vi "Write status_state.vi"(8 "error in (no error)":errorcluster, 10 "state":T1=enum."configure", 11 "MB_TCP in":refnum<class "MB_TCP.lvclass">) -> (0 "error out":errorcluster, 3 "MB_TCP out":refnum<class "MB_TCP.lvclass">)   [LabVIEW 2021, in "MB_TCP.lvclass"]
uses:
  MB_TCP.lvclass
  MB_TCP_State.ctl
  MB_TCP.lvclass/MB_TCP.ctl
  Eth Status/Eth Status.lvlib
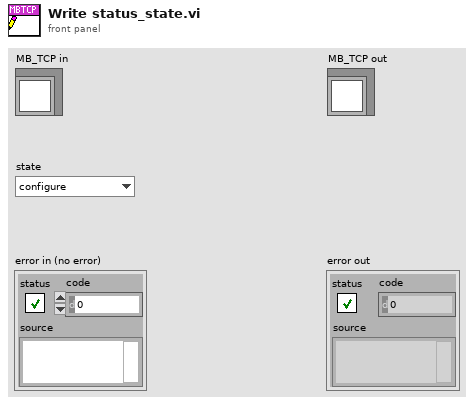
[diagram p1: front panel]
types:
  T1 = typedef "MB_TCP.lvclass/MB_TCP_State.ctl" = enum8{"initialization", "redefine", "standby", "connect", "wait to reconnect", "wait to reset timeout", "configure", "requests", "close connection", "stop"}
  T2 = typedef "Eth Status.lvlib/Status.ctl" = cluster{"Set_states":refnum<queue>[], "WrEn":refnum<data-value>, "errors":refnum<data-value>, "connect":refnum<data-value>, "state":refnum<data-value>}
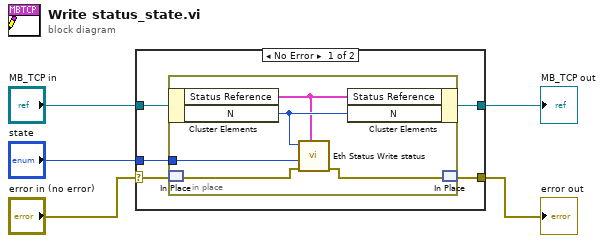
[diagram p0: block diagram]
diagram:
  n1 = case shown="No Error" "error in (no error)" {
    selector: "error in (no error)" -> [w8 w16]
    tunnel: [w6 w16] -> w3
    tunnel: [w7 w17] -> w4
    tunnel: "MB_TCP in" -> [w10 w17]
    tunnel: "state" -> [w9 _]
    frame No Error {
      n2 = in-place {
        in-place-border: w9 -> [w15]
        n3 = in-place-cluster #1(w10) -> ("Status Reference"=w11:T2, "N"=w12:i32)
        n4 = in-place-match #2(w8) -> (w14:errorcluster)
        n5 = call "Eth Status Write status.vi"("Status Reference"=w11, "error in (no error)"=w14, "status"=w15, "N"=w12) -> ("error out"=w13:errorcluster)  [unwired: 7 in]
        n6 = in-place-cluster #1("Status Reference"=w11, "N"=w12) -> (w7:refnum<class "MB_TCP.lvclass">)
        n7 = in-place-match #2(w13) -> (w6:errorcluster)
      }
    }
    frame Error {
    }
  }
  "error out" <- w3
  "MB_TCP out" <- w4
